vi "Continuous Measurement FPGA.vi"() -> ()   [LabVIEW 2014]
uses:
  <vilib>/Platform/TimedLoop/XDataNode/timing_clust.ctl
  <vilib>/Platform/TimedLoop/XDataNode/nitl_modes.ctl
  <vilib>/Platform/TimedLoop/XDataNode/wakeup.ctl
  <vilib>/rvi/Analysis/measure/FFT/simModelSupport/niFPGA FFT Streaming Sim Properties.ctl
  <vilib>/rvi/Analysis/measure/FFT/simModelSupport/niFPGA FFT Sim Stream Group Properties.ctl
  <vilib>/rvi/Analysis/measure/FFT/simModelSupport/niFPGA FFT Sim Types.ctl
  <vilib>/rvi/Analysis/measure/FFT/simModelSupport/niFpgaFFTSimArithmeticProperties.ctl
  <vilib>/rvi/Analysis/measure/FFT/simModelSupport/niFpgaFFTSimDfxp.ctl
  <vilib>/fxp/LVFixedPointQuantizationPolicyTypeDef.ctl
  <vilib>/rvi/Analysis/measure/FFT/XNode/niFpgaFFTButterflyDelays.ctl
  <vilib>/rvi/Emulation/niFpgaSctlEmulationGetInTimedLoop.vi
  <vilib>/rvi/Emulation/niFpgaEmulationReportErrorSimple.vi
  <vilib>/rvi/Emulation/niFpgaGetClockAttributes.vi
  <vilib>/rvi/Emulation/niFpgaCriticalErrorInLSC.vi
  <vilib>/rvi/Emulation/niFpgaEmulationIsFPGAContextNoSignature.vi
  <vilib>/rvi/errors/niFpgaSetErrorForExecOnDevCompSimple.vi
  <vilib>/rvi/eio/common/nirviEmuReportErrorAndStop.vi
  <vilib>/rvi/DataTransferAndStorage/Container/Common/niFpgaContainerGetUniqueNameForEmu.vi
  <vilib>/rvi/FIFO/Fifo_Resource/nirvififoEmulationSetSize.vi
  <vilib>/rvi/FIFO/Fifo_Resource/nirviFifoEmulationQueueMgr.vi
  <instcachedir>/0/nirviFifoEmulationQueueMgr_E5CAEC123FF24DC58D834DCA3CDAA9B5.lvgen/nirviFifoEmulationQueueMgr_E5CAEC123FF24DC58D834DCA3CDAA9B5_010.vi
  <vilib>/rvi/FIFO/Fifo_Resource/nirvififoEmulationCreateLock.vi
  <vilib>/rvi/Emulation/niFpgaProcessEmulError.vi
  <vilib>/rvi/FIFO/Fifo_Resource/nirvififoEmulationObtainLock.vi
  <vilib>/rvi/FIFO/Fifo_Resource/nirvififoEmulationReleaseLock.vi
  <vilib>/rvi/occurrence/nirviWaitOnOccurrenceBase.vi
  <vilib>/rvi/errors/nirviReportUnexpectedCaseInternalError.vi
  <vilib>/rvi/errors/nirviReportUnexpectedCaseInternalError (U32).vi
  <vilib>/rvi/FIFO/Fifo_Resource/nirvififoEmulationDetermineInputValidOut.vi
  <vilib>/rvi/Memory/Memory_Emulation/nirvimemoryFastEmulation.vi
  <vilib>/rvi/Memory/Memory_Emulation/nirvimemoryEmulation.vi
  <instcachedir>/0/nirviFifoEmulationQueueMgr_E5CAEC123FF24DC58D834DCA3CDAA9B5.lvgen/nirviFifoEmulationQueueMgr_E5CAEC123FF24DC58D834DCA3CDAA9B5_014.vi
  <vilib>/rvi/Memory/Memory_Emulation/niFpgaMemoryEmulationCacheClearOnFirstRun.vi
  <vilib>/rvi/Memory/Memory_Emulation/nirvimemoryEmulationManagerCache_MakeExclusive.vi
  <vilib>/rvi/Memory/Memory_Emulation/niFpgaMemoryEmulationValidateCache.vi
  <vilib>/rvi/Memory/Memory_Emulation/nirvimemoryEmulationManagerCache_InsertValue.vi
  <vilib>/Utility/error.llb/Clear Errors.vi
  <vilib>/rvi/Memory/Memory_Emulation/nirvimemoryEmulationManagerCache_ReleaseExclusive.vi
  <vilib>/rvi/Memory/Memory_Emulation/nirvimemoryEmulationManagerCache_GetValue.vi
  <vilib>/rvi/Memory/Memory_Emulation/nirvimemoryEmulationManagerCache_SetValue.vi
  <vilib>/rvi/Analysis/measure/FFT/simModelSupport/niFpgaFFTSimModelStreamingCore.vi
  <vilib>/rvi/eio/common/nirviEmuTemplateMethod_errors.vi
  <vilib>/Platform/TimedLoop/XDataNode/XDataNode.xnode
  <vilib>/rvi/DataTransferAndStorage/Container/XNode/niFpgaContainer.xnode
  <vilib>/rvi/FIFO/Fifo_Resource/nirvififoEmulationRead.vi
  <vilib>/rvi/FIFO/Fifo_Resource/nirvififoEmulationWrite.vi
  <vilib>/rvi/DataTransferAndStorage/Register/Emulation/niFpgaRegisterEmulation.vi
  <vilib>/rvi/FIFO/Fifo_Resource/nirvififoEmulationGetNumberOfElementsToWrite.vi
  <vilib>/rvi/Analysis/measure/FFT/XNode/niFpgaFFT.xnode
  <vilib>/eio/EIOMethodNode/EIOMethodNode.xnode
  <vilib>/Platform/TimedLoop/XDataNode/XDNodeRunTimeDep.lvlib
panel:
  in  "n-bit (2^(nbit) signals for Residual Extraction)":i32=8
  in  "Hanning window":bool=TRUE
  in  "First bin":i32=5
  in  "Last bin":i32=255
  in  "n":u32=5
  in  "Latency points":u32
  in  "lower limit 2":u32=682
  in  "lower limit 1":u32=57
  in  "upper limit 2":u32=1193
  in  "upper limit 1":u32=568
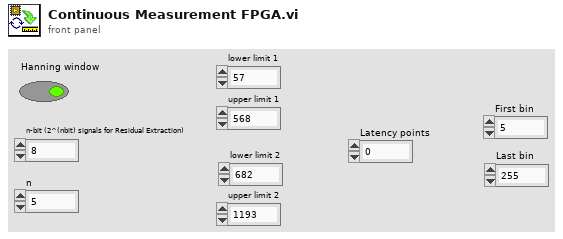
[diagram p1: front panel]
types:
  T1 = typedef "XDNodeRunTimeDep.lvlib/timing_clust.ctl" = cluster{"Expected End [f-1]":u64, "Actual End [f-1]":u64, "Finished Late? [f-1]":bool, "Expected End [i-1]":u64, "Actual End [i-1]":u64, "Finished Late? [i-1]":bool, "Expected Start [i]":u64, "Actual Start [i]":u64, "Expected Start [f]":u64, "Actual Start [f]":u64, "Source Name":string, "Structure Name":string, "Period":i64, "Deadline":i64, "Offset":i64, "Start":i64, "Priority":i32, "Timeout":i32, "Mode":T2, "Wakeup Reason":T3, "Error":errorcluster, "Source Type":string, "Secondary Source Type":string, "Global End Time":u64, "Global Start Time":u64, "Frame Duration":u64, "Iteration Duration":u64, "Assigned CPU":i32, "I/O Scan Engine Mode":u32}
  T2 = typedef "XDNodeRunTimeDep.lvlib/nitl_modes.ctl" = enum32{"No Change", "Process missed periods, maintain original phase", "Discard missed periods, maintain original phase", "Process missed periods, ignore original phase", "Discard missed periods, ignore original phase"}
  T3 = typedef "XDNodeRunTimeDep.lvlib/wakeup.ctl" = enum32{"Normal", "Aborted", "Asynchronous wakeup", "Timing source error", "Timed loop error", "Timeout"}
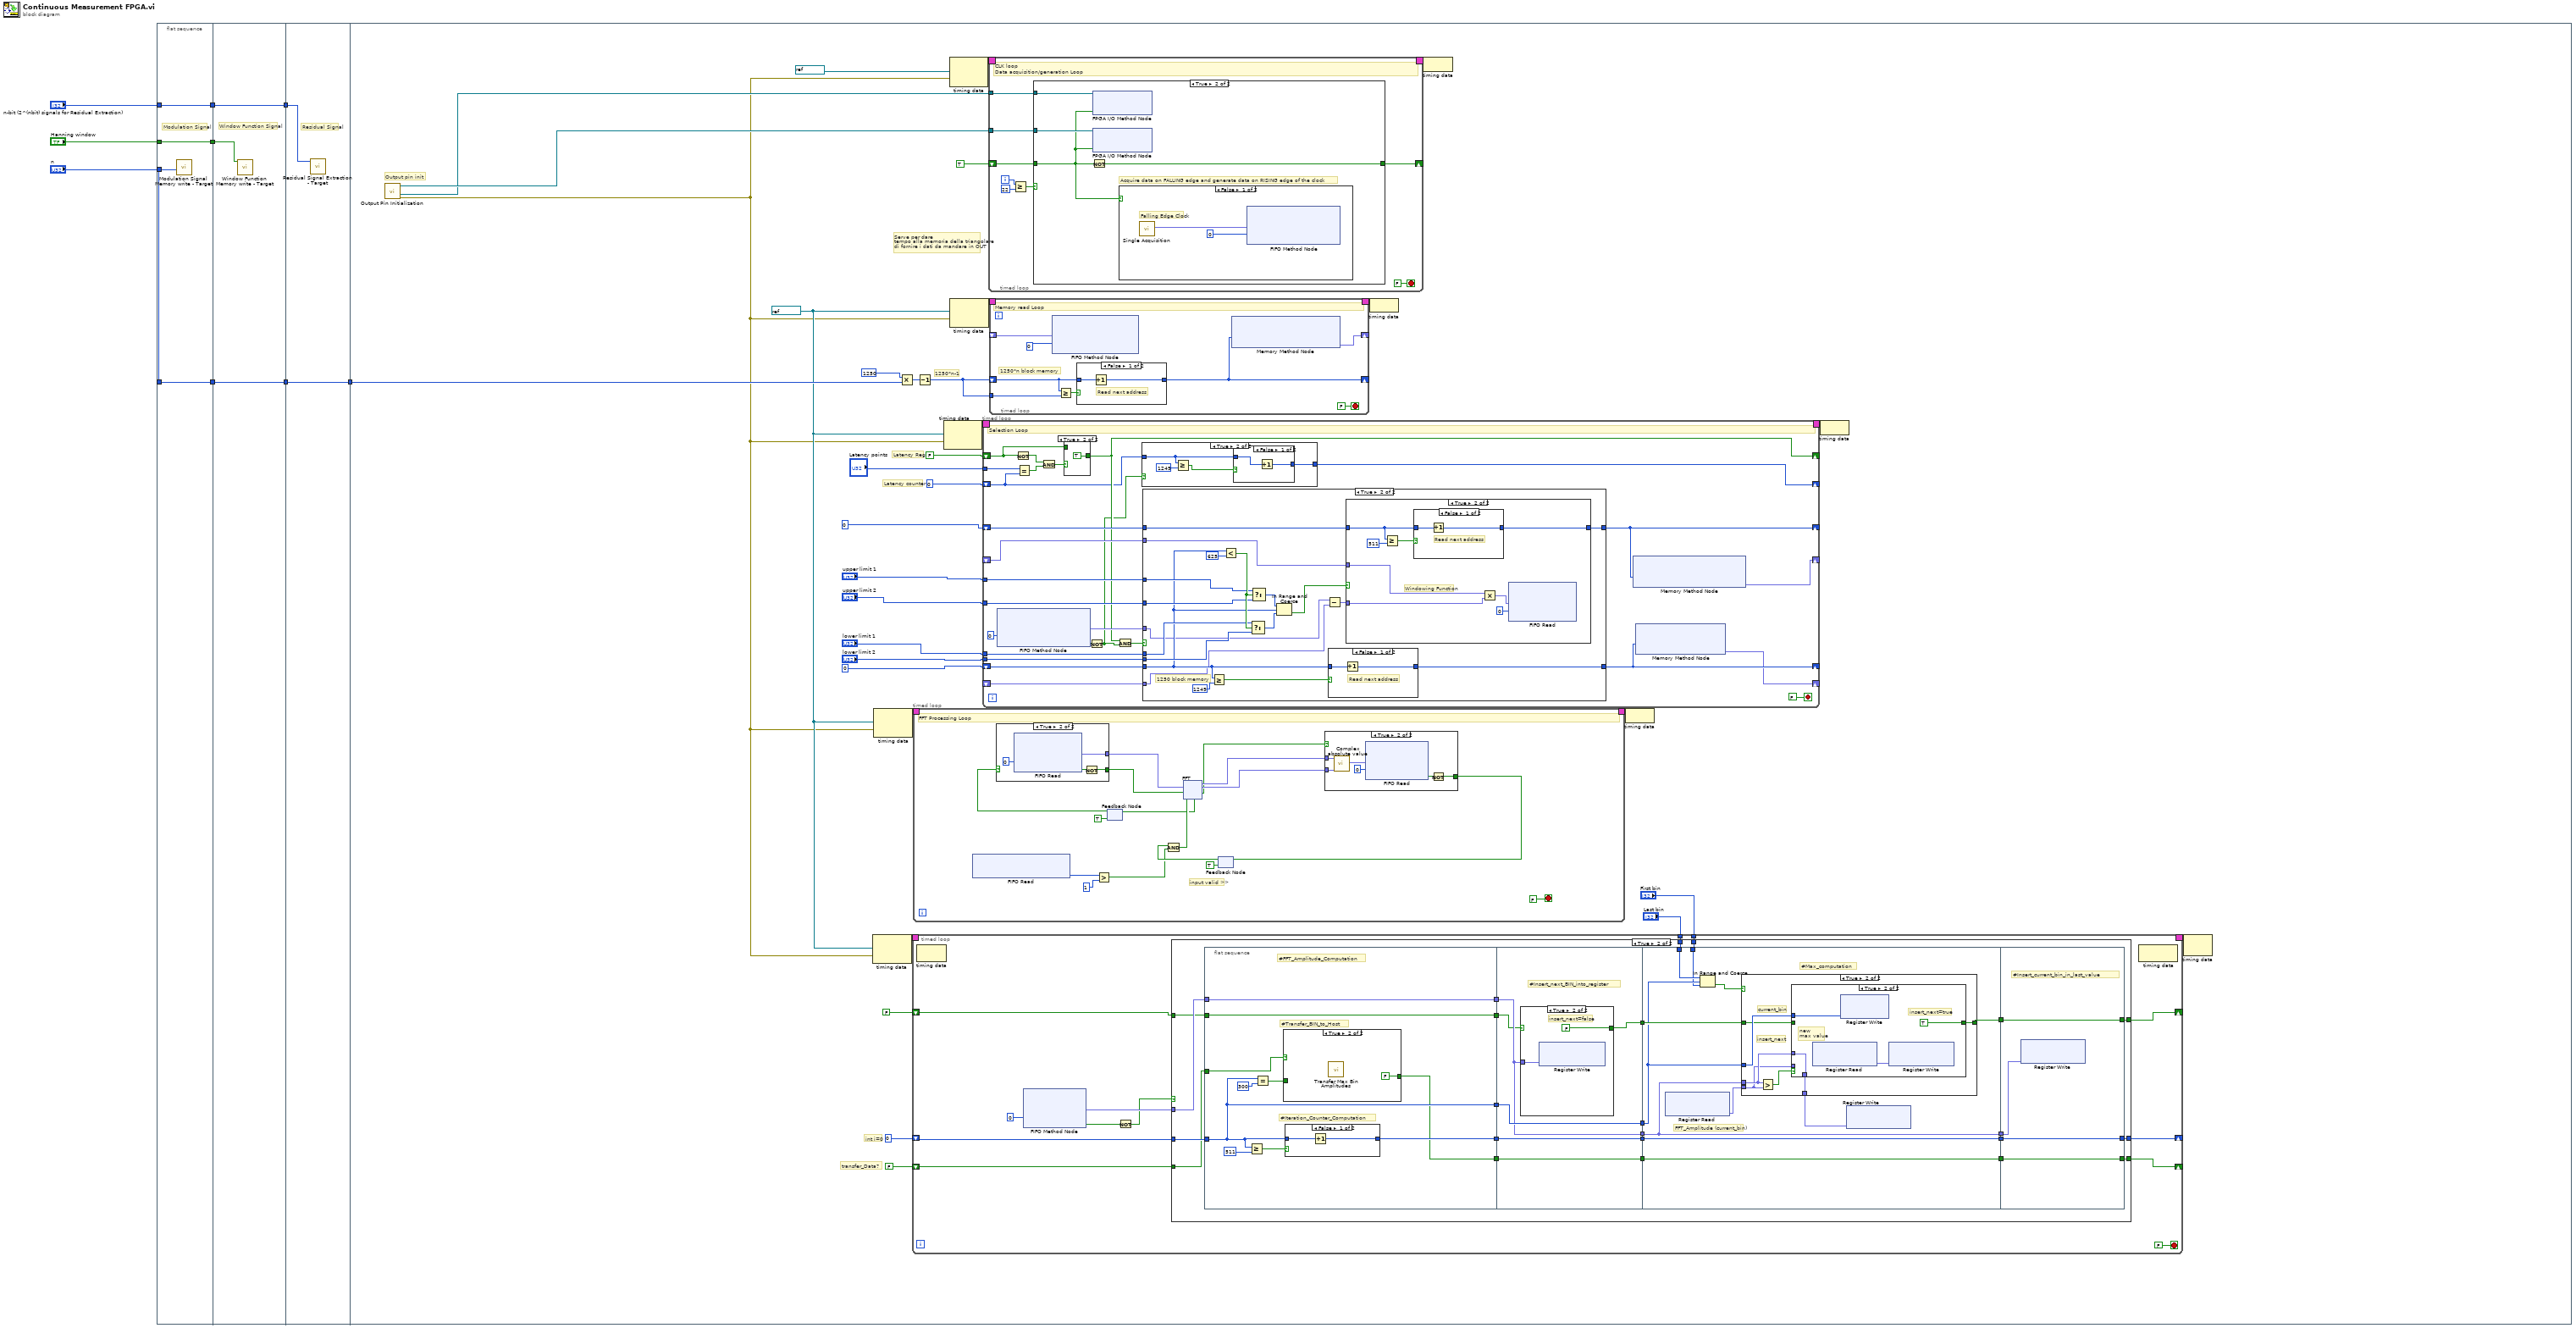
[diagram p0: block diagram]
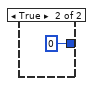
[diagram p3: hidden frame]
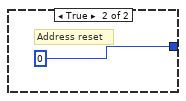
[diagram p7: hidden frame]
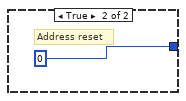
[diagram p8: hidden frame]
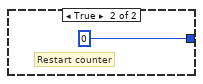
[diagram p11: hidden frame]
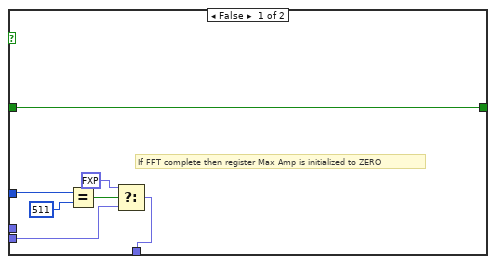
[diagram p13: hidden frame]
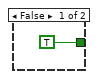
[diagram p15: hidden frame]
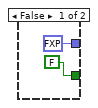
[diagram p16: hidden frame]
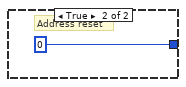
[diagram p17: hidden frame]
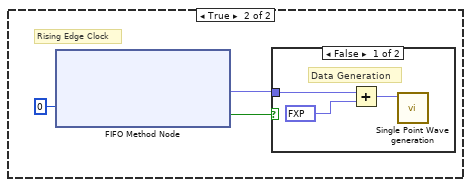
[diagram p19: hidden frame]
diagram:
  n1 = flat-sequence {
    tunnel: "n" -> [w13]
    tunnel: "n" -> [w12]
    tunnel: [w12] -> w8
    tunnel: "Hanning window" -> [w11]
    tunnel: [w11] -> w7
    tunnel: [w10] -> w3
    tunnel: "n-bit (2^(nbit) signals for Residual Extraction)" -> [w10]
    tunnel: w8 -> [w16]
    tunnel: [w16] -> w5
    tunnel: w7 -> [w15]
    tunnel: w3 -> [w14]
    tunnel: [w14] -> w1
    tunnel: w5 -> [w18]
    tunnel: [w18] -> w4
    tunnel: w1 -> [w17]
    tunnel: w4 -> [w39]
    frame #0 {
      # "Modulation Signal"
      n2 = call "Modulation Signal Memory write - Target.vi"("n"=w13) -> ()  [unwired: 11 in]
    }
    frame #1 {
      # "Window Function Signal"
      n3 = call "Window Function Memory write - Target.vi"("Hanning window"=w15) -> ()  [unwired: 11 in]
    }
    frame #2 {
      # "Residual Signal"
      n4 = call "Residual Signal Extraction - Target.vi"("n-bit (2^nbit medie)"=w17) -> ()  [unwired: 11 in]
    }
    frame #3 {
      w29 = refnum<k21> "30MHz" ("Source Name")
      # "transfer_Data?"
      # "int i=0"
      # "1250*n-1"
      # "Serve per dare\ntempo alla memoria della triangolare\ndi fornire i dati da mandare in OUT"
      # "Latency counter"
      # "Latency Reg"
      # "Output pin init"
      n5 = call "Output Pin Initialization.vi"() -> ("error out"=w28:errorcluster, "I/O Out Clock DAC (pin16)"=w43:refnum<k21>, "I/O Out Clock ADC (pin17)"=w44:refnum<k21>)  [unwired: 8 in]
      n6 = node-c288(w29, w28) -> (w38:T1)
      n7 = node-c288(w29, w28) -> (w48:T1)
      n8 = Multiply(x=u32 1250, y=w39) -> (x*y=w41:u32)
      n9 = timed-loop {
        shift-right: [w141] -> _
        shift-left: FALSE -> [w140]
        shift-right: [w139] -> _
        shift-left: 0 ("Timeout") -> [w142]
        shift-right: [w138] -> _
        shift-left: FALSE -> [w134]
        tunnel: "Last bin" -> [w136]
        tunnel: "First bin" -> [w135]
        timing: w38 -> [_]
        timing-out: [_] -> w37
        stop <- FALSE stop-if-true
        n10 = node-c288() -> ()  [unwired: 1 in, 1 out]
        n11 = xnode ("FIFO Method Node")("Timeout"=0) -> ("Element"=w143:fxp<+,44,44>, "Timed Out?"=w144:bool)  [unwired: 1 in, 1 out]
        n12 = Not(x=w144) -> (.not. x?=w137:bool)
        n13 = case shown="True" w137 {
          tunnel: w143 -> [_ w172]
          tunnel: w142 -> [w149 w170]
          tunnel: [w149 w157] -> w139
          tunnel: w140 -> [w148 w164]
          tunnel: [w148 w159] -> w141
          tunnel: w136 -> [_ w156]
          tunnel: w135 -> [_ w155]
          tunnel: w134 -> [w147 w154]
          tunnel: [w147 w153] -> w138
          frame False {
            # "Data are NOT ready in FIFO"
          }
          frame True {
            n14 = flat-sequence {
              tunnel: w172 -> [w173]
              tunnel: [w173] -> w171
              tunnel: w170 -> [w177]
              tunnel: [w182] -> w169
              tunnel: [w177] -> w166
              tunnel: [w179] -> w165
              tunnel: w164 -> [w179]
              tunnel: w154 -> [w176]
              tunnel: [w174] -> w152
              tunnel: w171 -> [w191]
              tunnel: w169 -> [w193]
              tunnel: [w193] -> w168
              tunnel: w166 -> [w192]
              tunnel: w165 -> [w189]
              tunnel: [w192] -> w163
              tunnel: [w191] -> w162
              tunnel: [w188] -> w161
              tunnel: w152 -> [w190]
              tunnel: [w190] -> w151
              tunnel: w168 -> [w207]
              tunnel: [w207] -> w167
              tunnel: w163 -> [w202]
              tunnel: w162 -> [w204]
              tunnel: w161 -> [w205]
              tunnel: [w204] -> w160
              tunnel: [w203] -> w158
              tunnel: w156 -> [w199]
              tunnel: w155 -> [w198]
              tunnel: w151 -> [w197]
              tunnel: [w197] -> w150
              tunnel: w167 -> [w229]
              tunnel: w160 -> [w231]
              tunnel: w158 -> [w230]
              tunnel: [w230] -> w159
              tunnel: [w229] -> w157
              tunnel: [w228] -> w153
              tunnel: w150 -> [w228]
              frame #0 {
                # "#Transfer_BIN_to_Host"
                # "#Iteration_Counter_Computation"
                # "#FFT_Amplitude_Computation"
                n15 = Greater Or Equal?(x=w177, y=511) -> (x >= y?=w180:bool)
                n16 = Equal?(x=w177, y=300) -> (x = y?=w175:bool)
                n17 = case shown="True" w176 {
                  tunnel: w175 -> [w183 _]
                  tunnel: [w183 FALSE] -> w174
                  frame False {
                    # "FFT Comp is NOT finished"
                  }
                  frame True {
                    n18 = call "Transfer Max Bin Amplitudes.vi"() -> ()  [unwired: 12 in]
                  }
                }
                n19 = case shown="False" w180 {
                  tunnel: w177 -> [w185 _]
                  tunnel: [w186 0 ("Timeout")] -> w182
                  frame False {
                    n20 = Increment(x=w185) -> (x+1=w186:i32)
                  }
                  frame True {
                    # "Restart counter"
                  }
                }
              }
              frame #1 {
                # "#Insert_next_BIN_into_register"
                n21 = case shown="True" w189 {
                  selector: w189 -> [w194 _]
                  tunnel: [w194 FALSE] -> w188
                  tunnel: w191 -> [_ w195]
                  frame False {
                  }
                  frame True {
                    # "insert_next=false"
                    n22 = xnode ("Register Write")("Data"=w195) -> ()  [unwired: 1 in, 1 out]
                  }
                }
              }
              frame #2 {
                # "FFT_Amplitude (current_bin)"
                # "#Max_computation"
                n23 = xnode ("Register Read")() -> ("Data"=w201:fxp<+,44,44>)  [unwired: 1 in, 1 out]
                n24 = In Range and Coerce(upper limit=w199, x=w202, lower limit=w198) -> (In Range?=w206:bool)  [unwired: 1 out]
                n25 = case shown="True" w206 {
                  tunnel: w204 -> [_ w220]
                  tunnel: w202 -> [w212 w219]
                  tunnel: w205 -> [w214 w218]
                  tunnel: [w214 w217] -> w203
                  tunnel: w201 -> [w210 w215]
                  tunnel: [w208 w216] -> w200
                  frame False {
                    # "If FFT complete then register Max Amp is initialized to ZERO"
                    n26 = Equal?(x=w212, y=511) -> (x = y?=w213:bool)
                    n27 = Select(t=fxp<+,44,44> 0.0, s=w213, f=w210) -> (s? t:f=w208:fxp<+,44,44>)
                  }
                  frame True {
                    # "insert_next"
                    # "current_bin"
                    n28 = Greater?(x=w220, y=w215) -> (0:w221:bool)
                    n29 = case shown="True" w221 {
                      tunnel: w220 -> [_ w225]
                      tunnel: w219 -> [_ w227]
                      tunnel: w218 -> [w223 _]
                      tunnel: [w223 TRUE] -> w217
                      tunnel: [w222 w225] -> w216
                      tunnel: w215 -> [w222 _]
                      frame False {
                        # "Old value is re-written"
                      }
                      frame True {
                        # "new\nmax value"
                        # "insert_next=true"
                        n30 = xnode ("Register Read")() -> ("Data"=w224:fxp<+,44,44>)  [unwired: 1 in, 1 out]
                        n31 = xnode ("Register Write")("Data"=w227) -> ()  [unwired: 1 in, 1 out]
                        n32 = xnode ("Register Write")("Data"=w224) -> ()  [unwired: 1 in, 1 out]
                      }
                    }
                  }
                }
                n33 = xnode ("Register Write")("Data"=w200) -> ()  [unwired: 1 in, 1 out]
              }
              frame #3 {
                # "#Insert_current_bin_in_last_value"
                n34 = xnode ("Register Write")("Data"=w231) -> ()  [unwired: 1 in, 1 out]
              }
            }
          }
        }
        n35 = node-c288() -> ()  [unwired: 1 in, 1 out]
      }
      n36 = timed-loop {
        timing: w48 -> [_]
        timing-out: [_] -> w47
        stop <- FALSE stop-if-true
        # "input valid >>"
        # "FFT Processing Loop"
        n37 = xnode ("FIFO Read")() -> ("Number of Elements to Write"=w237:u32)  [unwired: 1 in, 1 out]
        n38 = Greater?(x=w237, y=u32 1) -> (0:w238:bool)
        n39 = feedback #1(TRUE ("ready for input")) -> (w252:bool)
        n40 = case shown="True" w252 {
          tunnel: [FALSE w291] -> w242
          tunnel: [fxp<+/-,12,12> 0.0 ("Element") w288] -> w243
          frame False {
          }
          frame True {
            n41 = xnode ("FIFO Read")("Timeout"=0) -> ("Element"=w288:fxp<+/-,12,12>, "Timed Out?"=w290:bool)  [unwired: 1 in, 1 out]
            n42 = Not(x=w290) -> (.not. x?=w291:bool)
          }
        }
        n43 = feedback #2(TRUE) -> (w248:bool)
        n44 = Compound Arithmetic op=AND(w248, w238) -> (w247:bool)
        n45 = xnode "FFT"("real data in"=w243, "input valid"=w242, "ready for output"=w247) -> ("ready for input"=w246:bool, "real data out"=w245:fxp<+/-,22,22>, "imaginary data out"=w244:fxp<+/-,22,22>, "output valid"=w241:bool)  [unwired: 2 in, 1 out]
        n46 = feedback-in #1(w246) -> ()
        n47 = case shown="True" w241 {
          tunnel: w245 -> [_ w285]
          tunnel: w244 -> [_ w284]
          tunnel: [TRUE w283] -> w240
          frame False {
          }
          frame True {
            n48 = call "Complex absolute value.vi"("Im"=w284, "Re"=w285) -> ("Square Absolute Value"=w282:fxp<+,44,44>)  [unwired: 9 in]
            n49 = xnode ("FIFO Read")("Element"=w282, "Timeout"=0) -> ("Timed Out?"=w280:bool)  [unwired: 1 in, 1 out]
            n50 = Not(x=w280) -> (.not. x?=w283:bool)
          }
        }
        n51 = feedback-in #2(w240) -> ()
      }
      n52 = Decrement(x=w41) -> (x-1=w40:u32)
      n53 = node-c288(w29, w28) -> (w31:T1)
      n54 = node-c288(refnum<k21> "60MHz" ("Source Name"), w28) -> (w52:T1)
      n55 = node-c288(w29, w28) -> (w50:T1)
      n56 = timed-loop {
        timing: w31 -> [_]
        timing-out: [_] -> w30
        shift-right: [w54] -> _
        shift-left: u32 0 -> [w65]
        tunnel: "upper limit 1" -> [w74]
        tunnel: "upper limit 2" -> [w73]
        tunnel: "lower limit 1" -> [w72]
        tunnel: "lower limit 2" -> [w71]
        shift-right: [w67] -> _
        shift-left: u32 0 -> [w70]
        shift-right: [w68] -> _
        shift-left: _ -> [w69]
        shift-right: [w59] -> _
        shift-left: FALSE -> [w60]
        tunnel: "Latency points" -> [w64]
        shift-right: [w57] -> _
        shift-left: u32 0 -> [w56]
        shift-right: [w53] -> _
        shift-left: _ -> [w55]
        stop <- FALSE stop-if-true
        # "Selection Loop"
        n57 = xnode ("FIFO Method Node")("Timeout"=0) -> ("Element"=w76:fxp<+/-,12,12>, "Timed Out?"=w77:bool)  [unwired: 1 in, 1 out]
        n58 = Not(x=w60) -> (.not. x?=w63:bool)
        n59 = Equal?(x=w64, y=w56) -> (x = y?=w62:bool)
        n60 = And(x=w63, y=w62) -> (x .and. y?=w61:bool)
        n61 = case shown="True" w61 {
          tunnel: [w87 TRUE] -> w59
          tunnel: w60 -> [w87 _]
          frame False {
          }
          frame True {
          }
        }
        n62 = Not(x=w77) -> (.not. x?=w58:bool)
        n63 = And(x=w59, y=w58) -> (x .and. y?=w66:bool)
        n64 = case shown="True" w58 {
          tunnel: w56 -> [w79 w82]
          tunnel: [w79 w80] -> w57
          frame False {
          }
          frame True {
            n65 = Greater Or Equal?(x=w82, y=u32 1249) -> (x >= y?=w81:bool)
            n66 = case shown="False" w81 {
              tunnel: w82 -> [w85 _]
              tunnel: [w84 u32 0] -> w80
              frame False {
                n67 = Increment(x=w85) -> (x+1=w84:u32)
              }
              frame True {
              }
            }
          }
        }
        n68 = case shown="True" w66 {
          tunnel: [w90 w107] -> w54
          tunnel: w65 -> [w90 w95]
          tunnel: w76 -> [_ w92]
          tunnel: w74 -> [_ w102]
          tunnel: w73 -> [_ w101]
          tunnel: w72 -> [_ w100]
          tunnel: w71 -> [_ w99]
          tunnel: w70 -> [w89 w96]
          tunnel: [w89 w98] -> w67
          tunnel: w69 -> [_ w97]
          tunnel: w55 -> [_ w91]
          frame False {
          }
          frame True {
            # "1250 block memory"
            n69 = Greater Or Equal?(x=w95, y=u32 1249) -> (x >= y?=w108:bool)
            n70 = Less?(x=w95, y=u32 625) -> (x < y?=w103:bool)
            n71 = Select(t=w100, s=w103, f=w99) -> (s? t:f=w105:u32)
            n72 = Select(t=w102, s=w103, f=w101) -> (s? t:f=w106:u32)
            n73 = In Range and Coerce(upper limit=w106, x=w95, lower limit=w105) -> (In Range?=w94:bool)  [unwired: 1 out]
            n74 = Subtract(x=w92, y=w91) -> (x-y=w93:fxp<+/-,12,12>)
            n75 = case shown="False" w108 {
              tunnel: w95 -> [w123 _]
              tunnel: [w122 u32 0] -> w107
              frame False {
                # "Read next address"
                n76 = Increment(x=w123) -> (x+1=w122:u32)
              }
              frame True {
                # "Address reset"
              }
            }
            n77 = case shown="True" w94 {
              tunnel: w93 -> [_ w111]
              tunnel: w96 -> [w110 w116]
              tunnel: [w110 w118] -> w98
              tunnel: w97 -> [_ w114]
              frame False {
              }
              frame True {
                # "Windowing Function"
                n78 = Greater Or Equal?(x=w116, y=u32 511) -> (x >= y?=w117:bool)
                n79 = case shown="False" w117 {
                  tunnel: w116 -> [w120 _]
                  tunnel: [w119 u32 0] -> w118
                  frame False {
                    # "Read next address"
                    n80 = Increment(x=w120) -> (x+1=w119:u32)
                  }
                  frame True {
                    # "Address reset"
                  }
                }
                n81 = Multiply(x=w114, y=w111) -> (x*y=w112:fxp<+/-,12,12>)
                n82 = xnode ("FIFO Read")("Element"=w112, "Timeout"=0) -> ()  [unwired: 1 in, 2 out]
              }
            }
          }
        }
        n83 = xnode ("Memory Method Node")("Address"=w67) -> ("Data"=w68:fxp<+,8,1>)  [unwired: 1 in, 1 out]
        n84 = xnode ("Memory Method Node")("Address"=w54) -> ("Data"=w53:fxp<+/-,12,12>)  [unwired: 1 in, 1 out]
      }
      n85 = timed-loop {
        timing: w52 -> [_]
        timing-out: [_] -> w51
        shift-right: [w322] -> _
        shift-left: TRUE -> [w320]
        tunnel: w43 -> [w324]
        tunnel: w44 -> [w321]
        i -> [w318]
        stop <- FALSE stop-if-true
        # "CLK loop\nData acquisition/generation Loop"
        n86 = Greater Or Equal?(x=w318, y=22) -> (x >= y?=w317:bool)
        n87 = case shown="True" w317 {
          tunnel: w324 -> [_ w329]
          tunnel: [w325 w328] -> w322
          tunnel: w321 -> [_ w327]
          tunnel: w320 -> [w325 w326]
          frame False {
          }
          frame True {
            # "Acquire data on FALLING edge and generate data on RISING edge of the clock"
            n88 = Not(x=w326) -> (.not. x?=w328:bool)
            n89 = xnode "FPGA I/O Method Node"("FPGA I/O In"=w329, "Data"=w326) -> ()  [unwired: 1 out]
            n90 = xnode "FPGA I/O Method Node"("FPGA I/O In"=w327, "Data"=w326) -> ()  [unwired: 1 out]
            n91 = case shown="False" w326 {
              frame False {
                # "Falling Edge Clock"
                n92 = call "Single Acquisition.vi"() -> ("Out"=w331:fxp<+/-,12,12>)  [unwired: 10 in, 1 out]
                n93 = xnode ("FIFO Method Node")("Element"=w331, "Timeout"=0) -> ()  [unwired: 1 in, 2 out]
              }
              frame True {
                # "Rising Edge Clock"
                n94 = xnode ("FIFO Method Node")("Timeout"=0) -> ("Element"=w332:fxp<+/-,12,12>, "Timed Out?"=w333:bool)  [unwired: 1 in, 1 out]
                n95 = case shown="False" w333 {
                  tunnel: w332 -> [w337 _]
                  frame False {
                    # "Data Generation"
                    n96 = Add(x=w337, y=fxp<+,12,12> 2048.0) -> (x+y=w335:fxp<+/-,14,14>)
                    n97 = call "Single Point Wave generation.vi"("Data To Write"=w335) -> ()  [unwired: 10 in, 1 out]
                  }
                  frame True {
                    # "FPGA memory slow"
                  }
                }
              }
            }
          }
        }
      }
      n98 = timed-loop {
        timing: w50 -> [_]
        timing-out: [_] -> w49
        shift-right: [w300] -> _
        shift-left: w40 -> [w304]
        shift-right: [w302] -> _
        shift-left: _ -> [w301]
        tunnel: w40 -> [w299]
        stop <- FALSE stop-if-true
        # "1250*n block memory"
        # "Memory read Loop"
        n99 = xnode ("FIFO Method Node")("Element"=w301, "Timeout"=0) -> ()  [unwired: 1 in, 2 out]
        n100 = Greater Or Equal?(x=w304, y=w299) -> (x >= y?=w306:bool)
        n101 = case shown="False" w306 {
          tunnel: w304 -> [w308 _]
          tunnel: [w307 u32 0] -> w300
          frame False {
            # "Read next address"
            n102 = Increment(x=w308) -> (x+1=w307:u32)
          }
          frame True {
            # "Address reset"
          }
        }
        n103 = xnode ("Memory Method Node")("Address"=w300) -> ("Data"=w302:fxp<+/-,12,12>)  [unwired: 1 in, 1 out]
      }
      n104 = node-c288(w49) -> ()
      n105 = node-c288(w51) -> ()
      n106 = node-c288(w47) -> ()
      n107 = node-c288(w30) -> ()
      n108 = node-c288(w37) -> ()  [unwired: 1 out]
    }
  }
